vi "SendMessageAndWait.vi"(6 "timeout in ms (-1)":i32=-1, 8 "error in (no error)":errorcluster, 9 "PYTHON Node":T1, 10 "Argument String":string, 11 "PYTHON Command":string) -> (0 "error out":errorcluster, 3 "Reply":T2)   [LabVIEW 2013, in "JKI_Python_Bridge_for_LV.lvlib" / "Server.lvclass"]
uses:
  Server.lvclass
  Type Definitions/Python Response - Cluster.ctl
  Type Definitions/Python Node.ctl
  CallHandler/PyObject.lvclass
  Call/Call.lvclass
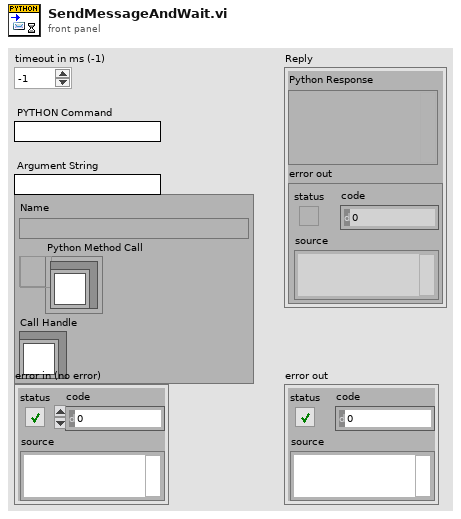
[diagram p1: front panel]
types:
  T1 = typedef "JKI_Python_Bridge_for_LV.lvlib/Server.lvclass/Python Node.ctl" = cluster{"Name":string, "Python Method Call":refnum<user-event>, "Call Handle":refnum<class "PyObject.lvclass">}
  T2 = typedef "JKI_Python_Bridge_for_LV.lvlib/Server.lvclass/Python Response - Cluster.ctl" = cluster{"Python Response":variant, "error out":errorcluster}
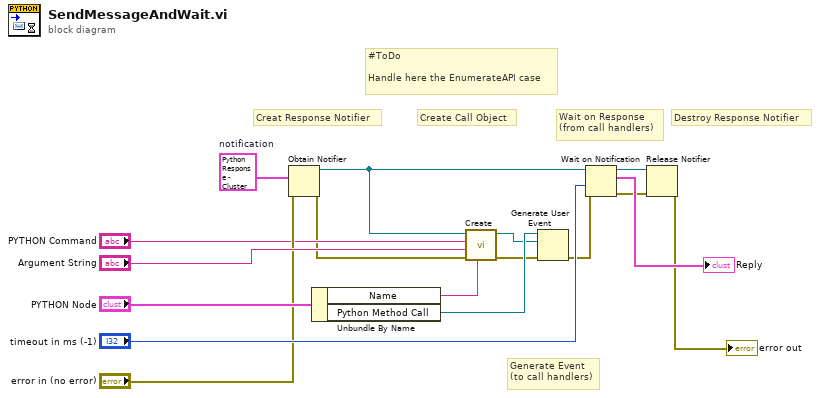
[diagram p0: block diagram]
diagram:
  w3 = T2 {"Python Response"=variant, "error out"={"status"=FALSE, "code"=0, "source"=""}}  # notification
  # "Creat Response Notifier"
  # "Create Call Object"
  # "Destroy Response Notifier"
  # "Wait on Response\n(from call handlers)"
  # "Generate Event\n(to call handlers)"
  # "#ToDo\n\nHandle here the EnumerateAPI case"
  n1 = Obtain Notifier(notification data type=w3, error in (no error)="error in (no error)") -> (notifier out=w8:refnum<notifier>, error out=w6:errorcluster)  [unwired: 1 in, 2 out]
  n2 = Unbundle By Name("PYTHON Node") -> ("Name"=w1:string, "Python Method Call"=w10:refnum<user-event>)
  n3 = call "Create.vi"("Object Name"=w1, "error in (no error)"=w6, "Arguments"="Argument String", "Method Name"="PYTHON Command", "Response Notifier"=w8) -> ("error out"=w7:errorcluster, "Call out"=w9:refnum<class "Call.lvclass">)  [unwired: 5 in]
  n4 = Generate User Event(user event=w10, event data cluster=w9, error in=w7) -> (error out=w2:errorcluster)  [unwired: 1 in, 1 out]
  n5 = Wait on Notification(notifier=w8, timeout in ms (-1)="timeout in ms (-1)", error in (no error)=w2) -> (notifier out=w4:refnum<notifier>, notification=→"Reply":T2, error out=w5:errorcluster)  [unwired: 2 out]
  n6 = Release Notifier(notifier=w4, error in (no error)=w5) -> (error out=→"error out":errorcluster)  [unwired: 3 out]
